vi "写入-企业信息.vi"(8 "error in (no error)":errorcluster caption="错误输入（无错误）", 10 "企业信息":T1, 11 "PC个人客户端输入":refnum<class "PC个人客户端.lvclass">) -> (0 "error out":errorcluster caption="错误输出", 3 "PC个人客户端输出":refnum<class "PC个人客户端.lvclass">)   [LabVIEW 2013, in "PC个人客户端.lvclass"]
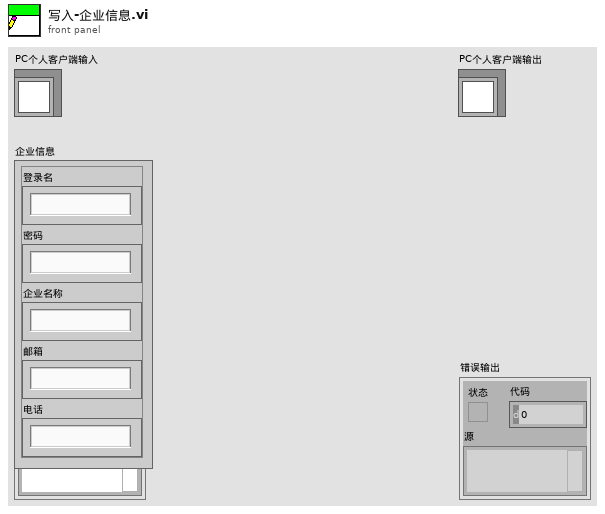
[diagram p1: front panel]
types:
  T1 = cluster{"登录名":string, "密码":string, "企业名称":string, "邮箱":string, "电话":string}
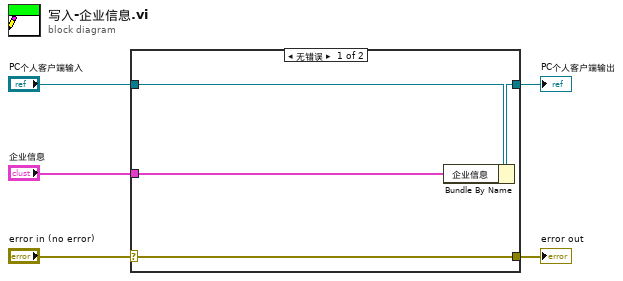
[diagram p0: block diagram]
diagram:
  n1 = case shown="无错误" "error in (no error)" {
    selector: "error in (no error)" -> [w9 w10]
    tunnel: [w9 w10] -> w4
    tunnel: [w7 w11] -> w2
    tunnel: "PC个人客户端输入" -> [w8 w11]
    tunnel: "企业信息" -> [w6 _]
    frame No Error {
      n2 = Bundle By Name(cluster=w8, "企业信息"=w6) -> (w7:refnum<class "PC个人客户端.lvclass">)
    }
    frame Error {
    }
  }
  "error out" <- w4
  "PC个人客户端输出" <- w2
